vi "Output_UI.vi"(7 "OutputDetails":T2, 8 "error in":errorcluster, 9 "Functionality":T1=enum."SendAcknowledgement", 10 "Testbench":bool=TRUE, 11 "SMEnqueuer":refnum<class "Message Enqueuer.lvclass">) -> (0 "error out":errorcluster)   [LabVIEW 2019, in "ZenGage v3.0 UI.lvclass"]
uses:
  ZenGage v3.0 UI.lvclass
  <vilib>/ActorFramework/Message Enqueuer/Message Priority.ctl
  <vilib>/ActorFramework/Message Enqueuer/Message Enqueuer.lvclass
  Inspection Statemachine/Inspection Statemachine Messages/ErrorMessage_SM Msg/ErrorMessage_SM Msg.lvclass
  Inspection Statemachine/Inspection Statemachine Messages/SelectedPart_SM Msg/SelectedPart_SM Msg.lvclass
  Inspection Statemachine/Inspection Statemachine Messages/Acknowledgement_SM Msg/Acknowledgement_SM.lvclass
  Inspection Statemachine/Inspection Statemachine Messages/InitiateCamOpticsDiagnostics_SM Msg/InitiateCamOpticsDiagnostics_SM Msg.lvclass
  Inspection Statemachine/Inspection Statemachine Messages/InitiateSensorDiagnostics_SM Msg/InitiateSensorDiagnostics_SM Msg.lvclass
  Inspection Statemachine/Inspection Statemachine Messages/ActionOnPopup_SM Msg/ActionOnPopup_SM.lvclass
  Inspection Statemachine/Inspection Statemachine Messages/EventReason_SM Msg/EventReason_SM Msg.lvclass
  Inspection Statemachine/Inspection Statemachine Messages/IgnoredFailCountDetails_SM Msg/IgnoredFailCountDetails_SM Msg.lvclass
  Inspection Statemachine/Inspection Statemachine Messages/ButtonPressed_SM Msg/ButtonPressed_SM Msg.lvclass
  Common/Controls/Acknowledgement.ctl
  Type Definitions/General/OutputDetails.ctl
  Type Definitions/General/Output choice.ctl
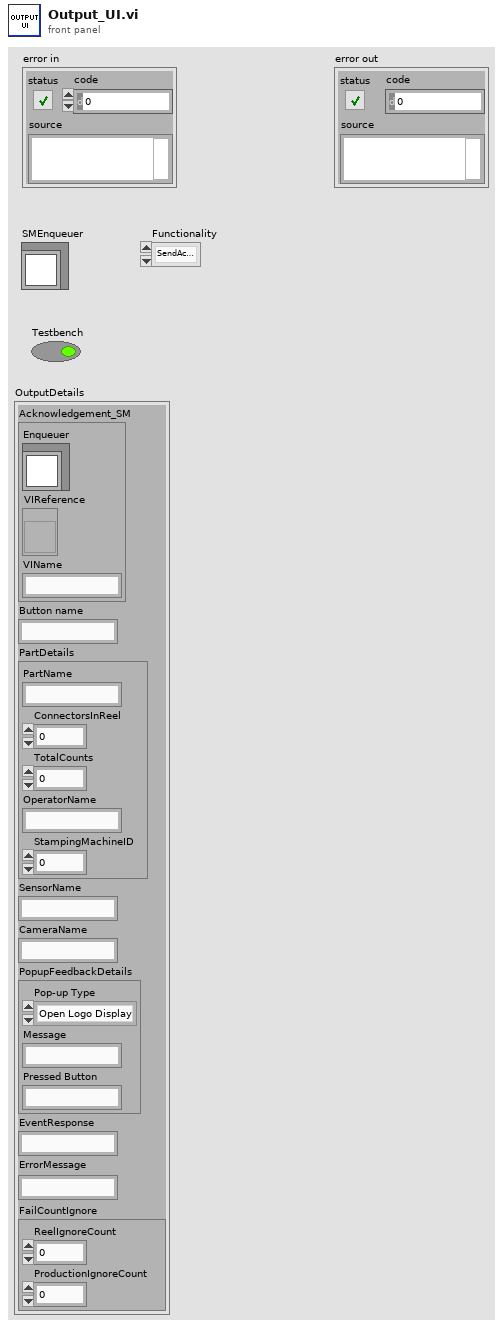
[diagram p1: front panel]
types:
  T1 = typedef "ZenGage v3.0 UI.lvclass/Output choice.ctl" = enum16{"SendIgnoredFailCount", "SendPartDetails", "ButtonPress", "SendAcknowledgement", "InitiateCameraDiagnostics", "InitiateSensorDiagnostics", "SendPopupResponse", "SendEventReasonResponse", "SendErrorDetails"}
  T2 = typedef "ZenGage v3.0 UI.lvclass/OutputDetails.ctl" = cluster{"Acknowledgement_SM":T3, "Button name":string, "PartDetails":cluster{"PartName":string, "ConnectorsInReel":u64, "TotalCounts":u64, "OperatorName":string, "StampingMachineID":u32}, "SensorName":string, "CameraName":string, "PopupFeedbackDetails":cluster{"Pop-up Type":enum16{"Open Logo Display", "Close Logo Display", "Open Loading Bar", "Close Loading Bar", "Open Alert Display", "Close Alert Display", "One button dialog box", "Two button dialog box", "User Authentication"}, "Message":string, "Pressed Button":string}, "EventResponse":string, "ErrorMessage":string, "FailCountIgnore":cluster{"ReelIgnoreCount":u64, "ProductionIgnoreCount":u64}}
  T3 = typedef "Acknowledgement.ctl" = cluster{"Enqueuer":refnum<class "Message Enqueuer.lvclass">, "VIReference":refnum<vi>, "VIName":string}
  T4 = typedef "Actor Framework.lvlib/Message Enqueuer.lvclass/Message Priority.ctl" = enum16{"Low", "Normal", "High"}
  T5 = cluster{"Pop-up Type":enum16{"Open Logo Display", "Close Logo Display", "Open Loading Bar", "Close Loading Bar", "Open Alert Display", "Close Alert Display", "One button dialog box", "Two button dialog box", "User Authentication"}, "Message":string, "Pressed Button":string}
  T6 = cluster{"PartName":string, "ConnectorsInReel":u64, "TotalCounts":u64, "OperatorName":string, "StampingMachineID":u32}
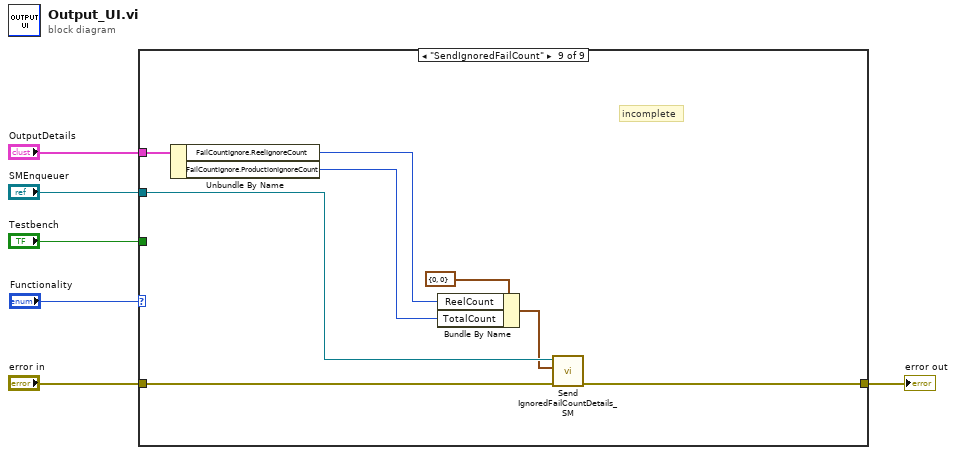
[diagram p0: block diagram]
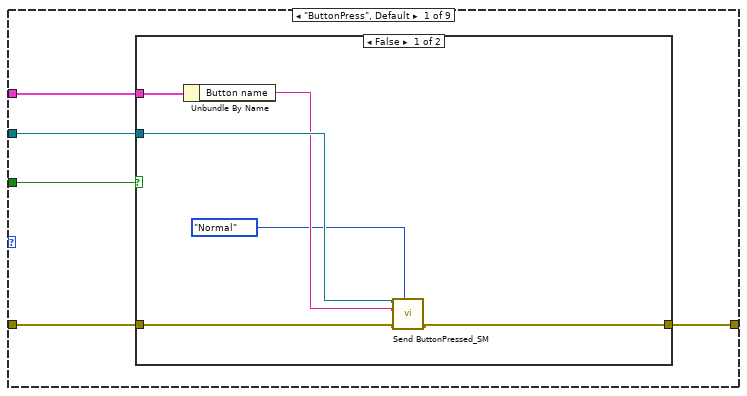
[diagram p2: hidden frame]
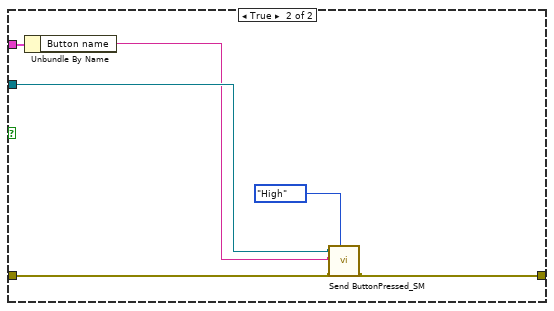
[diagram p3: hidden frame]
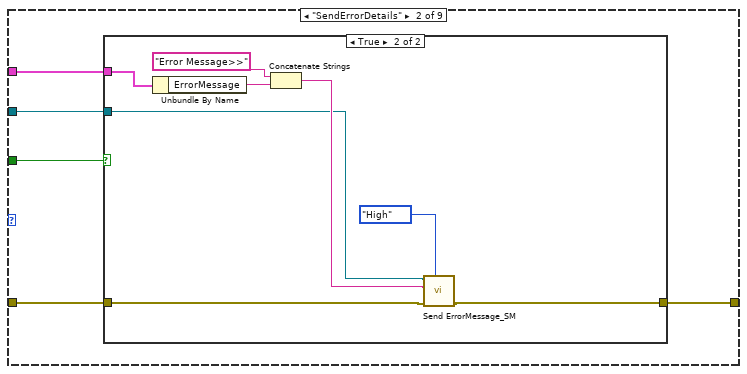
[diagram p4: hidden frame]
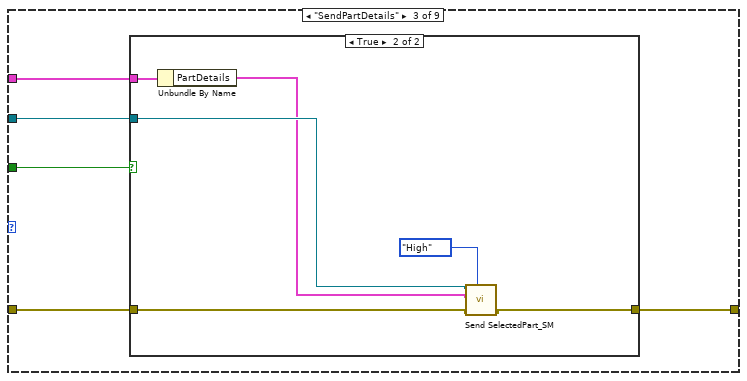
[diagram p6: hidden frame]
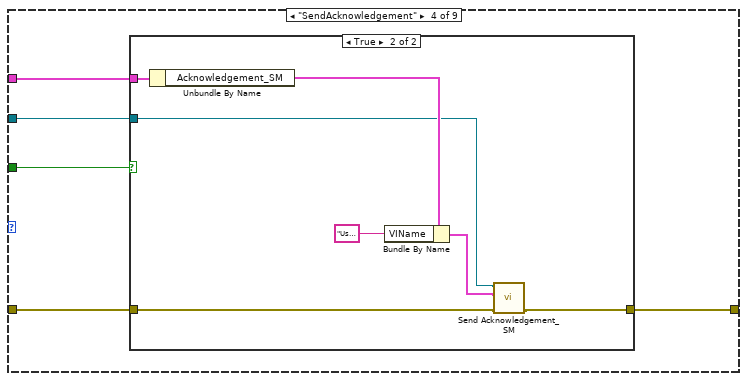
[diagram p8: hidden frame]
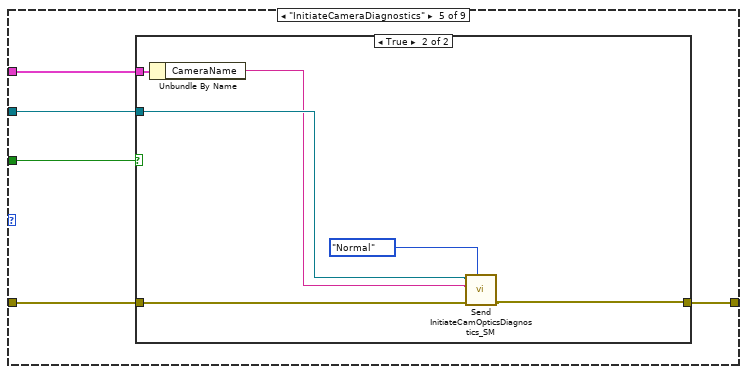
[diagram p10: hidden frame]
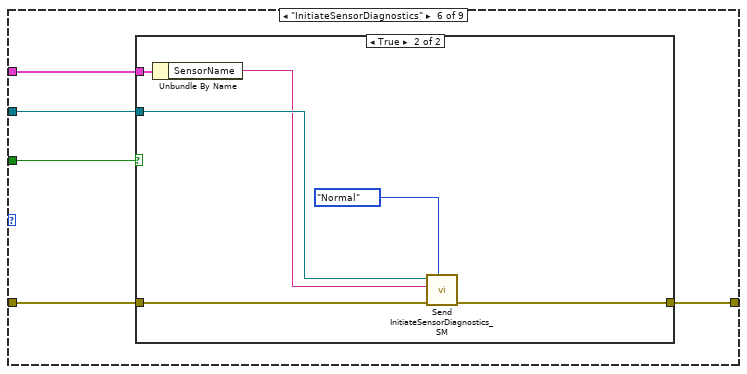
[diagram p12: hidden frame]
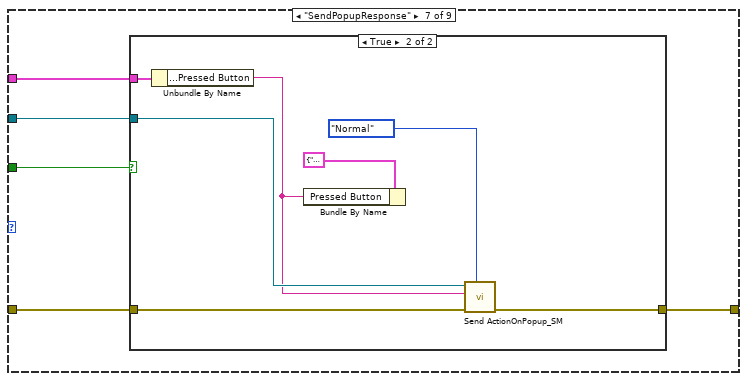
[diagram p14: hidden frame]
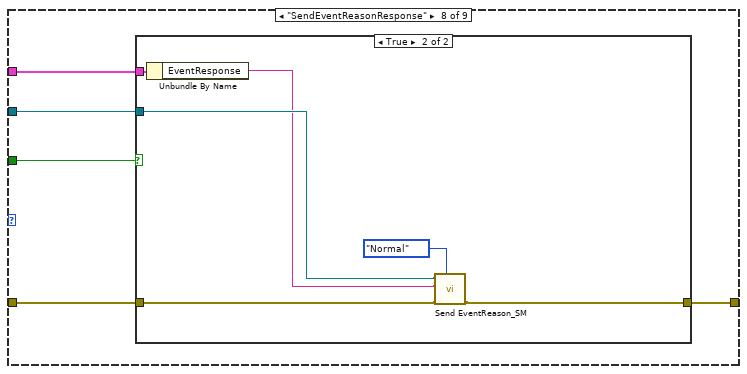
[diagram p16: hidden frame]
diagram:
  n1 = case shown="\"SendIgnoredFailCount\"" "Functionality" {
    tunnel: "SMEnqueuer" -> [w9 w26 w40 w52 w65 w77 w89 w102 w117]
    tunnel: "error in" -> [w10 w27 w41 w53 w66 w78 w90 w103 w119]
    tunnel: "Testbench" -> [w11 w28 w42 w54 w67 w79 w91 w104 _]
    tunnel: [w8 w25 w39 w51 w64 w76 w88 w101 w118] -> w2
    tunnel: "OutputDetails" -> [w7 w24 w38 w50 w63 w75 w87 w100 w116]
    frame "ButtonPress", Default {
      n2 = case shown="False" w11 {
        tunnel: w10 -> [w16 w22]
        tunnel: w9 -> [w14 w20]
        tunnel: [w15 w21] -> w8
        tunnel: w7 -> [w17 w23]
        frame False {
          n3 = Unbundle By Name(w17) -> ("Button name"=w13:string)
          n4 = call "Send ButtonPressed_SM.vi"("Message Priority (Normal)"=Message_Priority."Normal", "error in (no error)"=w16, "ButtonPress"=w13, "Message Enqueuer"=w14) -> ("error out"=w15:errorcluster)  [unwired: 6 in, 1 out]
        }
        frame True {
          n5 = Unbundle By Name(w23) -> ("Button name"=w19:string)
          n6 = call "Send ButtonPressed_SM.vi"("Message Priority (Normal)"=Message_Priority."High", "error in (no error)"=w22, "ButtonPress"=w19, "Message Enqueuer"=w20) -> ("error out"=w21:errorcluster)  [unwired: 6 in, 1 out]
        }
      }
    }
    frame "SendErrorDetails" {
      n7 = case shown="True" w28 {
        tunnel: w27 -> [w29 w34]
        tunnel: w26 -> [_ w31]
        tunnel: [w29 w33] -> w25
        tunnel: w24 -> [_ w37]
        frame False {
        }
        frame True {
          n8 = Unbundle By Name(w37) -> ("ErrorMessage"=w36:string)
          n9 = Concatenate Strings("Error Message>>", w36) -> (w32:string)
          n10 = call "Send ErrorMessage_SM.vi"("Message Priority (Normal)"=Message_Priority."High", "error in (no error)"=w34, "Error Message"=w32, "Message Enqueuer"=w31) -> ("error out"=w33:errorcluster)  [unwired: 6 in, 1 out]
        }
      }
    }
    frame "SendPartDetails" {
      n11 = case shown="True" w42 {
        tunnel: w41 -> [w43 w48]
        tunnel: w40 -> [_ w46]
        tunnel: [w43 w47] -> w39
        tunnel: w38 -> [_ w49]
        frame False {
        }
        frame True {
          n12 = Unbundle By Name(w49) -> ("PartDetails"=w45:T6)
          n13 = call "Send SelectedPart_SM.vi"("Message Priority (Normal)"=Message_Priority."High", "error in (no error)"=w48, "SelectedPart"=w45, "Message Enqueuer"=w46) -> ("error out"=w47:errorcluster)  [unwired: 6 in, 1 out]
        }
      }
    }
    frame "SendAcknowledgement" {
      n14 = case shown="True" w54 {
        tunnel: w53 -> [w55 w59]
        tunnel: w52 -> [_ w57]
        tunnel: [w55 w58] -> w51
        tunnel: w50 -> [_ w62]
        frame False {
        }
        frame True {
          n15 = Unbundle By Name(w62) -> ("Acknowledgement_SM"=w61:T3)
          n16 = Bundle By Name(cluster=w61, "VIName"="User Interface") -> (w56:T3)
          n17 = call "Send Acknowledgement_SM.vi"("error in (no error)"=w59, "Acknowledgement"=w56, "Message Enqueuer"=w57) -> ("error out"=w58:errorcluster)  [unwired: 7 in, 1 out]
        }
      }
    }
    frame "InitiateCameraDiagnostics" {
      n18 = case shown="True" w67 {
        tunnel: w66 -> [w68 w73]
        tunnel: w65 -> [_ w71]
        tunnel: [w68 w72] -> w64
        tunnel: w63 -> [_ w74]
        frame False {
        }
        frame True {
          n19 = Unbundle By Name(w74) -> ("CameraName"=w70:string)
          n20 = call "Send InitiateCamOpticsDiagnostics_SM.vi"("Message Priority (Normal)"=Message_Priority."Normal", "error in (no error)"=w73, "CameraName"=w70, "Message Enqueuer"=w71) -> ("error out"=w72:errorcluster)  [unwired: 6 in, 1 out]
        }
      }
    }
    frame "InitiateSensorDiagnostics" {
      n21 = case shown="True" w79 {
        tunnel: w78 -> [w80 w85]
        tunnel: w77 -> [_ w83]
        tunnel: [w80 w84] -> w76
        tunnel: w75 -> [_ w86]
        frame False {
        }
        frame True {
          n22 = Unbundle By Name(w86) -> ("SensorName"=w82:string)
          n23 = call "Send InitiateSensorDiagnostics_SM.vi"("Message Priority (Normal)"=Message_Priority."Normal", "error in (no error)"=w85, "Sensor name"=w82, "Message Enqueuer"=w83) -> ("error out"=w84:errorcluster)  [unwired: 6 in, 1 out]
        }
      }
    }
    frame "SendPopupResponse" {
      n24 = case shown="True" w91 {
        tunnel: w90 -> [w92 w97]
        tunnel: w89 -> [_ w94]
        tunnel: [w92 w96] -> w88
        tunnel: w87 -> [_ w99]
        frame False {
        }
        frame True {
          n25 = Unbundle By Name(w99) -> ("PopupFeedbackDetails.Pressed Button"=w93:string)
          n26 = Bundle By Name(cluster=T5 {"Pop-up Type"=enum."Open Logo Display", "Message"="", "Pressed Button"=""} ("PopupFeedbackDetails"), "Pressed Button"=w93) -> ()  [unwired: 1 out]
          n27 = call "Send ActionOnPopup_SM.vi"("Message Priority (Normal)"=Message_Priority."Normal", "error in (no error)"=w97, "Action on Popup"=w93, "Message Enqueuer"=w94) -> ("error out"=w96:errorcluster)  [unwired: 6 in, 1 out]
        }
      }
    }
    frame "SendEventReasonResponse" {
      n28 = case shown="True" w104 {
        tunnel: w103 -> [w105 w110]
        tunnel: w102 -> [_ w108]
        tunnel: [w105 w109] -> w101
        tunnel: w100 -> [_ w111]
        frame False {
        }
        frame True {
          n29 = Unbundle By Name(w111) -> ("EventResponse"=w107:string)
          n30 = call "Send EventReason_SM.vi"("Message Priority (Normal)"=Message_Priority."Normal", "error in (no error)"=w110, "EventReason"=w107, "Message Enqueuer"=w108) -> ("error out"=w109:errorcluster)  [unwired: 6 in, 1 out]
        }
      }
    }
    frame "SendIgnoredFailCount" {
      # "incomplete"
      n31 = Unbundle By Name(w116) -> ("FailCountIgnore.ReelIgnoreCount"=w113:u64, "FailCountIgnore.ProductionIgnoreCount"=w112:u64)
      n32 = Bundle By Name(cluster=cluster{"ReelCount":u64, "TotalCount":u64} {"ReelCount"=0, "TotalCount"=0} ("IgnoredCountDetails"), "ReelCount"=w113, "TotalCount"=w112) -> (w114:cluster{"ReelCount":u64, "TotalCount":u64})
      n33 = call "Send IgnoredFailCountDetails_SM.vi"("error in (no error)"=w119, "IgnoredCountDetails"=w114, "Message Enqueuer"=w117) -> ("error out"=w118:errorcluster)  [unwired: 7 in, 1 out]
    }
  }
  "error out" <- w2
